vi "Translator.Enum.WriteStrings.vi"(8 "error out":errorcluster, 10 "Strings":string[](array[string]), 11 "idx":i32) -> (0 "error out 2":errorcluster)   [LabVIEW 2016]
uses:
  EventLog/EventLog.Buffer.Action.ctl
  Translator.Global.vi
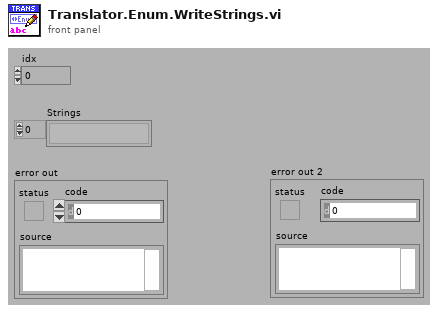
[diagram p1: front panel]
types:
  T1 = typedef "EventLog.Buffer.Action.ctl" = enum16{"init", "re-init", "clear", "set translator", "translate", "add", "get"}
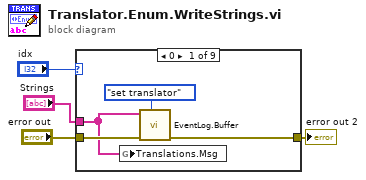
[diagram p0: block diagram]
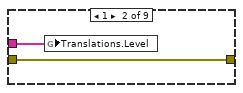
[diagram p2: hidden frame]
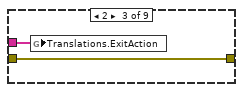
[diagram p3: hidden frame]
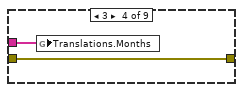
[diagram p4: hidden frame]
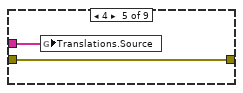
[diagram p5: hidden frame]
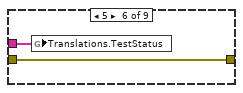
[diagram p6: hidden frame]
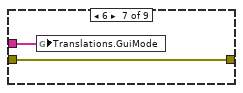
[diagram p7: hidden frame]
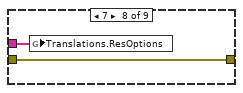
[diagram p8: hidden frame]
diagram:
  n1 = case shown="0" "idx" {
    tunnel: "Strings" -> [w5 w10 w12 w14 w16 w18 w20 w22 _]
    tunnel: "error out" -> [w8 w9 w11 w13 w15 w17 w19 w21 w23]
    tunnel: [w7 w9 w11 w13 w15 w17 w19 w21 w23] -> w2
    frame 0 {
      n2 = global write "Translator.Global.vi" "Translations.Msg"(w5) -> ()
      n3 = call "EventLog.Buffer.vi"("action (get)"=EventLog.Buffer.Action."set translator" ("action (read)"), "error in"=w8, "Translations"=w5) -> ("error out"=w7:errorcluster)  [unwired: 5 in, 3 out]
    }
    frame 1 {
      n4 = global write "Translator.Global.vi" "Translations.Level"(w10) -> ()
    }
    frame 2 {
      n5 = global write "Translator.Global.vi" "Translations.ExitAction"(w12) -> ()
    }
    frame 3 {
      n6 = global write "Translator.Global.vi" "Translations.Months"(w14) -> ()
    }
    frame 4 {
      n7 = global write "Translator.Global.vi" "Translations.Source"(w16) -> ()
    }
    frame 5 {
      n8 = global write "Translator.Global.vi" "Translations.TestStatus"(w18) -> ()
    }
    frame 6 {
      n9 = global write "Translator.Global.vi" "Translations.GuiMode"(w20) -> ()
    }
    frame 7 {
      n10 = global write "Translator.Global.vi" "Translations.ResOptions"(w22) -> ()
    }
    frame Default {
    }
  }
  "error out 2" <- w2
